vi "Prep_Motors_Global.vi"(1 "B-Axis":refnum<k7>, 2 "Error In":errorcluster, 3 "Z-Axis":refnum<k7>, 4 "Y-Axis":refnum<k7>, 5 "X-Axis":refnum<k7>) -> (0 "Error Out":errorcluster)   [LabVIEW 2016]
uses:
  Utility/Global_Stage.vi
panel:
  in  "S/N B-Axis":i32=94865857
  in  "S/N Y-Axis":i32=83860202
  in  "S/N X-Axis":i32=83855365
  in  "S/N Z-Axis":i32=83860012
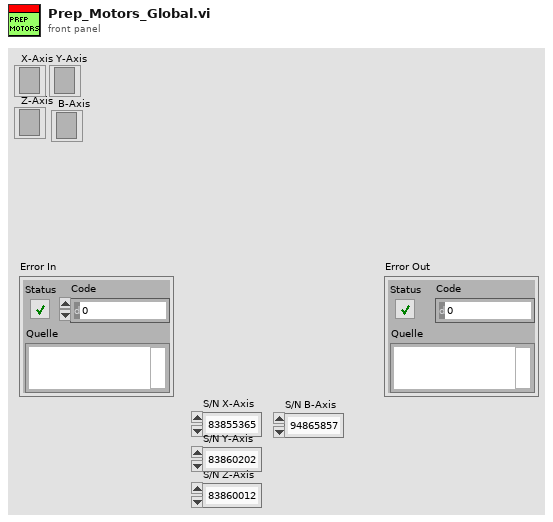
[diagram p1: front panel]
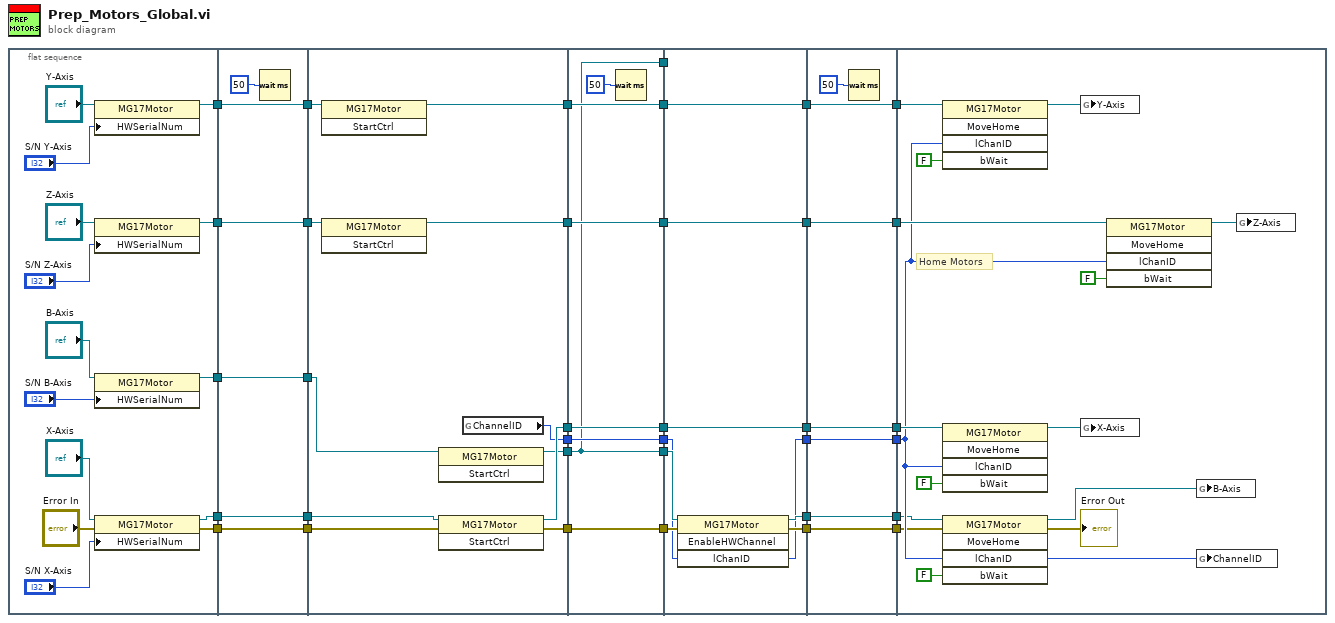
[diagram p0: block diagram]
diagram:
  n1 = flat-sequence {
    tunnel: [w49] -> w10
    tunnel: [w48] -> w8
    tunnel: [w47] -> w6
    tunnel: [w37] -> w4
    tunnel: [w36] -> w2
    tunnel: w10 -> [w55]
    tunnel: [w55] -> w9
    tunnel: w8 -> [w54]
    tunnel: [w54] -> w7
    tunnel: w6 -> [w53]
    tunnel: [w53] -> w5
    tunnel: w4 -> [w52]
    tunnel: [w52] -> w3
    tunnel: w2 -> [w51]
    tunnel: [w51] -> w1
    tunnel: [w66] -> w32
    tunnel: [w65] -> w33
    tunnel: [w64] -> w34
    tunnel: w9 -> [w63]
    tunnel: w7 -> [w62]
    tunnel: w5 -> [w61]
    tunnel: w3 -> [w60]
    tunnel: w1 -> [w59]
    tunnel: [w56] -> w35
    tunnel: [w58] -> w31
    tunnel: [w57] -> w30
    tunnel: w35 -> [w73]
    tunnel: [w73] -> w29
    tunnel: w34 -> [w72]
    tunnel: [w72] -> w28
    tunnel: w33 -> [w71]
    tunnel: [w71] -> w27
    tunnel: w32 -> [w70]
    tunnel: [w70] -> w26
    tunnel: w31 -> [w69]
    tunnel: [w69] -> w25
    tunnel: w30 -> [w67]
    tunnel: [w67] -> w24
    tunnel: [w67] -> w23
    tunnel: w29 -> [w79]
    tunnel: [w78] -> w22
    tunnel: w28 -> [w82]
    tunnel: [w82] -> w20
    tunnel: w27 -> [w81]
    tunnel: [w81] -> w18
    tunnel: w26 -> [w80]
    tunnel: [w80] -> w16
    tunnel: w25 -> [w75]
    tunnel: [w74] -> w14
    tunnel: w24 -> [_]
    tunnel: [w76] -> w12
    tunnel: w23 -> [w77]
    tunnel: w22 -> [w89]
    tunnel: [w89] -> w21
    tunnel: w20 -> [w88]
    tunnel: [w88] -> w19
    tunnel: w18 -> [w87]
    tunnel: [w87] -> w17
    tunnel: w16 -> [w86]
    tunnel: [w86] -> w15
    tunnel: w14 -> [w85]
    tunnel: [w85] -> w13
    tunnel: w12 -> [w84]
    tunnel: [w84] -> w11
    tunnel: w21 -> [w91]
    tunnel: w19 -> [w100]
    tunnel: w17 -> [w101]
    tunnel: w15 -> [w102]
    tunnel: w13 -> [w92]
    tunnel: w11 -> [w90]
    frame #0 {
      n2 = property on="Eigenschaftsknoten" class="MG17Motor"(reference="Y-Axis", "HWSerialNum"="S/N Y-Axis") -> (reference out=w48:refnum<k7>)  [unwired: 1 in, 1 out]
      n3 = property on="Eigenschaftsknoten" class="MG17Motor"(reference="Z-Axis", "HWSerialNum"="S/N Z-Axis") -> (reference out=w47:refnum<k7>)  [unwired: 1 in, 1 out]
      n4 = property on="Eigenschaftsknoten" class="MG17Motor"(reference="B-Axis", "HWSerialNum"="S/N B-Axis") -> (reference out=w37:refnum<k7>)  [unwired: 1 in, 1 out]
      n5 = property on="Eigenschaftsknoten" class="MG17Motor"(reference="X-Axis", error in="Error In", "HWSerialNum"="S/N X-Axis") -> (reference out=w49:refnum<k7>, error out=w36:errorcluster)
    }
    frame #1 {
      n6 = Wait (ms)(milliseconds to wait=u32 50) -> ()  [unwired: 1 out]
    }
    frame #2 {
      n7 = invoke class="MG17Motor" method="StartCtrl"(reference=w62) -> (reference out=w65:refnum<k7>)  [unwired: 2 in, 2 out]
      n8 = invoke class="MG17Motor" method="StartCtrl"(reference=w61) -> (reference out=w64:refnum<k7>)  [unwired: 2 in, 2 out]
      n9 = invoke class="MG17Motor" method="StartCtrl"(reference=w60) -> (reference out=w57:refnum<k7>)  [unwired: 2 in, 2 out]
      n10 = invoke class="MG17Motor" method="StartCtrl"(reference=w63, error in=w59) -> (reference out=w66:refnum<k7>, error out=w56:errorcluster)  [unwired: 1 in, 1 out]
      n11 = global read "Global_Stage.vi" "ChannelID"() -> (w58:i32)
    }
    frame #3 {
      n12 = Wait (ms)(milliseconds to wait=u32 50) -> ()  [unwired: 1 out]
    }
    frame #4 {
      n13 = invoke class="MG17Motor" method="EnableHWChannel"(reference=w77, error in=w79, "lChanID"=w75) -> (reference out=w76:refnum<k7>, error out=w78:errorcluster, "lChanID"=w74:i32)  [unwired: 1 in, 1 out]
    }
    frame #5 {
      n14 = Wait (ms)(milliseconds to wait=u32 50) -> ()  [unwired: 1 out]
    }
    frame #6 {
      # "Home Motors"
      n15 = invoke class="MG17Motor" method="MoveHome"(reference=w101, "lChanID"=w92, "bWait"=FALSE) -> (reference out=w98:refnum<k7>)  [unwired: 2 in, 4 out]
      n16 = invoke class="MG17Motor" method="MoveHome"(reference=w102, "lChanID"=w92, "bWait"=FALSE) -> (reference out=w99:refnum<k7>)  [unwired: 2 in, 4 out]
      n17 = invoke class="MG17Motor" method="MoveHome"(reference=w90, error in=w91, "lChanID"=w92, "bWait"=FALSE) -> (reference out=w95:refnum<k7>, error out=→"Error Out":errorcluster, "lChanID"=w93:i32)  [unwired: 1 in, 2 out]
      n18 = global write "Global_Stage.vi" "Y-Axis"(w98) -> ()
      n19 = global write "Global_Stage.vi" "X-Axis"(w99) -> ()
      n20 = invoke class="MG17Motor" method="MoveHome"(reference=w100, "lChanID"=w92, "bWait"=FALSE) -> (reference out=w97:refnum<k7>)  [unwired: 2 in, 4 out]
      n21 = global write "Global_Stage.vi" "B-Axis"(w95) -> ()
      n22 = global write "Global_Stage.vi" "ChannelID"(w93) -> ()
      n23 = global write "Global_Stage.vi" "Z-Axis"(w97) -> ()
    }
  }
